vi "Open Actor Core.vi"(8 "error in (no error)":errorcluster, 9 "Core Index (0)":i32, 10 "Actor's Self Q":refnum<class "Message Enqueuer.lvclass">, 11 "Monitor Data":refnum<class "Monitor Data.lvclass">) -> (0 "error out":errorcluster, 2 "Actor Core VI":string)   [LabVIEW 2017, in "MGI-Monitored Actor Core.lvlib" / "Monitor Data.lvclass"]
doc: "Opens the running Actor Core instance for the actor.\n\nIf called in the runtime environoment the Front Panel of the actor core may not be present, so this VI will throw an error.\n\nCopyright: MGI 2016\nAuthor: Derek Trepanier"
uses:
  Monitor Data.lvclass
  <vilib>/ActorFramework/Message Enqueuer/Message Enqueuer.lvclass
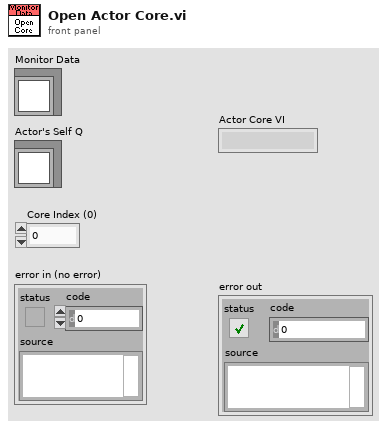
[diagram p1: front panel]
types:
  T1 = typedef "MGI-Monitored Actor Core.lvlib/Monitor Data.lvclass/Actor Data.ctl" = cluster{"Actor Type":string, "Actor Cores":string[], "Self":refnum<class "Message Enqueuer.lvclass">, "Caller":refnum<class "Message Enqueuer.lvclass">, "Actor Label":string, "Last Ping":dbl}
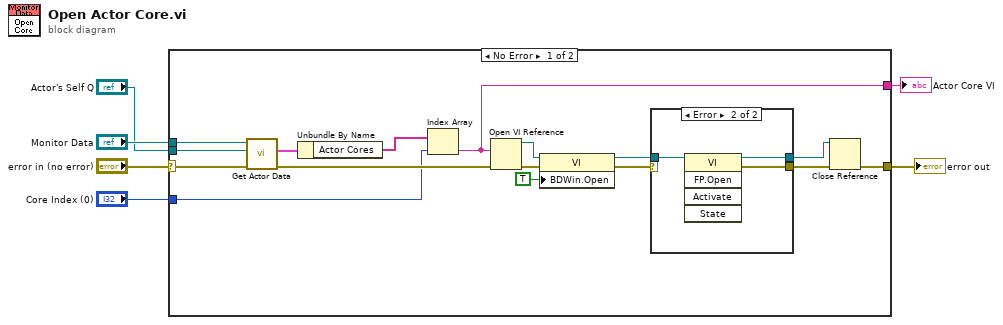
[diagram p0: block diagram]
diagram:
  n1 = case shown="No Error" "error in (no error)" {
    selector: "error in (no error)" -> [w10 w28]
    tunnel: "Monitor Data" -> [w22 _]
    tunnel: "Actor's Self Q" -> [w21 _]
    tunnel: [w12 w28] -> w4
    tunnel: [w8 _] -> w2
    tunnel: "Core Index (0)" -> [w7 _]
    frame No Error {
      n2 = call "Get Actor Data.vi"("error in (no error)"=w10, "Actor's Self Q"=w21, "Monitor Data in"=w22) -> ("error out"=w19:errorcluster, "Actor Data"=w20:T1)  [unwired: 5 in, 2 out]
      n3 = Unbundle By Name(w20) -> ("Actor Cores"=w9:string[])
      n4 = Index Array(array=w9, index=w7) -> (element=w8:string)
      n5 = Open VI Reference(vi path=w8, error in (no error)=w19) -> (vi reference=w18:refnum<vi>, error out=w17:errorcluster)  [unwired: 4 in]
      n6 = property class="VI"(reference=w18, error in=w17, "BDWin.Open"=TRUE ("Block Diagram Window:Open")) -> (reference out=w16:refnum<vi>, error out=w15:errorcluster)
      n7 = case shown="Error" w15 {
        selector: w15 -> [w24 _]
        tunnel: w16 -> [w23 w27]
        tunnel: [w23 w26] -> w11
        tunnel: [w24 w25] -> w13
        frame No Error {
        }
        frame Error {
          n8 = invoke class="VI" method="FP.Open"(reference=w27) -> (reference out=w26:refnum<vi>, error out=w25:errorcluster)  [unwired: 4 in, 3 out]
        }
      }
      n9 = Close Reference(reference=w11, error in (no error)=w13) -> (error out=w12:errorcluster)
    }
    frame Error {
    }
  }
  "error out" <- w4
  "Actor Core VI" <- w2
